vi "LoadAllPersistentData.vi"(8 "ErrorIn":errorcluster) -> (0 "ErrorOut":errorcluster)   [LabVIEW 2021, in "Application.lvclass"]
uses:
  Application.lvclass
  Interface_TAF_IApplicationConfiguration/IApplicationConfiguration/IApplicationConfiguration.lvclass
  Interface_TAF_ITAFObject/ITAFObject/ITAFObject.lvclass
  025b7748-fce9-48d0-88d4-1eb01e8d8b65.vi
  ce5b3271-6dfa-4a7e-af59-08ad89dcf7ac.vi
  a83cf28d-3d5c-43a3-b080-66f150894b72.vi
  <vilib>/TriekselSoft/TracerLibrary/TracerLibrary/Tracer/protected/SendMessage.vi
  <vilib>/TriekselSoft/TracerLibrary/TracerLibrary/Tracer/protected/Timestamp.vi
  a83cf28d-3d5c-43a3-b080-66f150894b72.vi/f75db090-0877-4668-94fb-75c2140b1617.vi
  <vilib>/TriekselSoft/TracerLibrary/TracerLibrary/Tracer/Tracer_Level-Debug.vi
  <vilib>/TriekselSoft/TracerLibrary/TracerLibrary/Tracer/protected/Tracer_ClassAttributes.vi
  Application_GetInstance.vi
  <vilib>/Utility/LVClass/Get LV Class Name.vi
  <vilib>/JDP Science/JSONtext/Variant to JSON Text.vi
  <vilib>/JDP Science/JSONtext/LVClass Serializer/JSONtext LVClass Serializer.lvclass
  Application.lvclass/Application.ctl
  C:/Localdata/Projects/TriekselSoft/TriekselsoftApplicationFramework/Source/.Externals/Interface_TAF_IApplicationConfiguration/IApplicationConfiguration/IApplicationConfiguration.lvclass
  C:/Localdata/Projects/TriekselSoft/TriekselsoftApplicationFramework/Source/IInterface/IInterface.lvclass
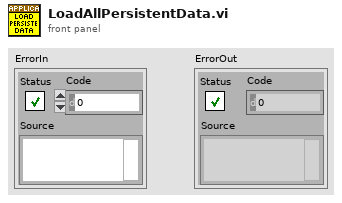
[diagram p1: front panel]
types:
  T1 = cluster{"Name":string, "ErrorOut":errorcluster, "DataOut":variant}
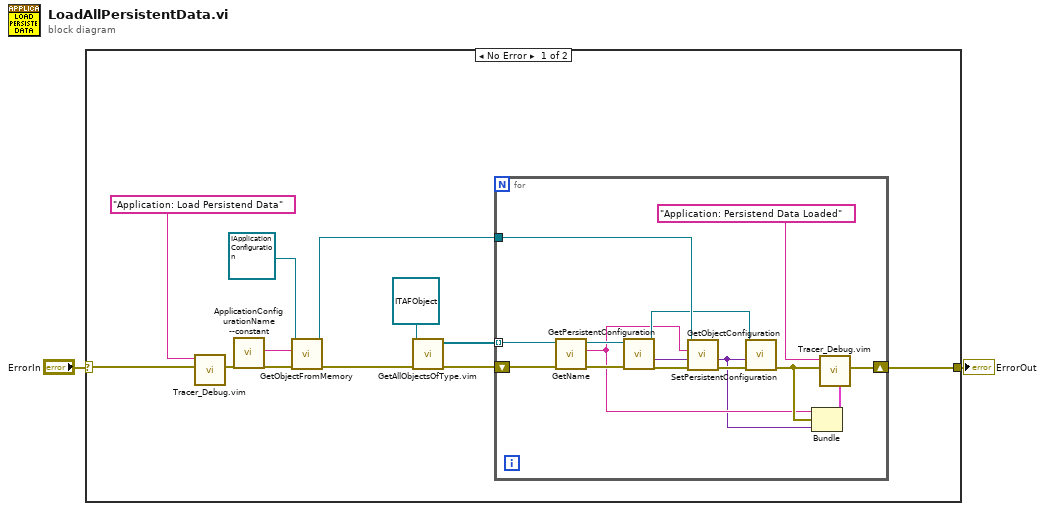
[diagram p0: block diagram]
diagram:
  n1 = case shown="No Error" "ErrorIn" {
    selector: "ErrorIn" -> [w9 w29]
    tunnel: [w11 w29] -> w1
    frame No Error {
      n2 = call "Tracer_Debug.vim"("error in (no error)"=w9, "Text"="Application: Load Persistend Data") -> ("error out"=w10:errorcluster)  [unwired: 9 in]
      n3 = call "ApplicationConfigurationName --constant.vi"() -> ("AppConfigName"=w7:string)  [unwired: 10 in, 1 out]
      n4 = call "GetObjectFromMemory.vi"("ErrorIn"=w10, "ObjectName"=w7, "Type"=refnum<class "IApplicationConfiguration.lvclass"> refnum ("IApplicationStructure")) -> ("ErrorOut"=w13:errorcluster, "ObjectOut"=w4:refnum<class "IApplicationConfiguration.lvclass">)  [unwired: 7 in]
      n5 = call "GetAllObjectsOfType.vim"("error in (no error)"=w13, "ObjectType"=refnum<class "ITAFObject.lvclass"> refnum ("NamedCreator")) -> ("error out"=w12:errorcluster, "ObjectsOut"=w5:refnum<class "ITAFObject.lvclass">[])  [unwired: 8 in]
      n6 = for {
        tunnel: w5 -> [w20] mode=indexing
        tunnel: w4 -> [w22]
        shift-right: [w23] -> w11
        shift-left: w12 -> [w28]
        n7 = call-dynamic "GetName.vi"("ErrorIn"=w28, "ObjectIn"=w20) -> ("ErrorOut"=w26:errorcluster, "Name"=w17:string, "ObjectOut"=w19:refnum<class "ITAFObject.lvclass">)  [unwired: 7 in]
        n8 = call-dynamic "GetPersistentConfiguration.vi"("ErrorIn"=w26, "ObjectIn"=w19) -> ("ErrorOut"=w27:errorcluster, "DataOut"=w21:variant, "ObjectOut"=w18:refnum<class "ITAFObject.lvclass">)  [unwired: 7 in]
        n9 = call-dynamic "GetObjectConfiguration.vi"("ErrorIn"=w27, "DataIn"=w21, "Label"=w17, "IApplicationStructureIn"=w22) -> ("ErrorOut"=w25:errorcluster, "DataOut"=w15:variant)  [unwired: 5 in, 1 out]
        n10 = call-dynamic "SetPersistentConfiguration.vi"("ErrorIn"=w25, "DataIn"=w15, "ObjectIn"=w18) -> ("ErrorOut"=w24:errorcluster)  [unwired: 6 in, 2 out]
        n11 = Bundle("Name"=w17, "ErrorOut"=w24, "DataOut"=w15) -> (w16:T1)  [unwired: 1 in]
        n12 = call "Tracer_Debug.vim"("Data"=w16, "error in (no error)"=w24, "Text"="Application: Persistend Data Loaded") -> ("error out"=w23:errorcluster)  [unwired: 8 in]
      }
    }
    frame Error {
    }
  }
  "ErrorOut" <- w1
